vi "SetUpDigi 12bit.vi"(6 "Therapy (T)":bool, 7 "Therapy VISA session in":refnum<visa-resource-name>, 8 "33250(T)/33120(F)":bool=TRUE, 10 "Trigger\nDC (T) AC (F)":bool, 11 "Acqiris ID":u32) -> (0 "Waveform\nGraph":cluster{i32, dbl, dbl[]}(graph), 1 "Equivalent RT delay\ndistance (mm)":dbl=1.5 format="%.4f", 2 "RF data Out":T3 {"Delay (micro s)" format="%.2f"}, 3 "Vert Settings":cluster{u16, i32, "Coupling":u16})   [LabVIEW 2022 SP3]
uses:
  Motion Controllers/-MotionRoutines/MotionGlobals.vi
  <vilib>/Analysis/NI_AALPro.lvlib
  <vilib>/Utility/file.llb/Write To Spreadsheet File (DBL).vi
  <vilib>/Analysis/NI_AALBase.lvlib
  <vilib>/Analysis/baseanly.llb/Mean (DBL).vi
panel:
  in  "LeCroy Path":u16(ring) items=["Pan T/R", "Pan Rec", "Miteq"]
  in  "Cytec T/R":u32
  in  "Panametrics P/R?":bool=TRUE
  in  "Board ID":T1=1 min=1 max=32 step=1
  in  "Save trace?":bool
  out "Lines in burst":i32=1 min=1 max=50000 step=1
  in  "cycles (f), time(t)":bool=TRUE
  in  "Set Panametrics":bool
  out "Total Delay (ms)":dbl=1.5 format="%.2f"
  in  "go to scan type":bool
  in  "Therapy Burst Set Up":T2={"Therapy Set Up"={"Burst time (ms)"=1.0, "Frequency (MHz)"=1.0, "Amplitude (mV)"=10.0}, "Divide prf by"=1, "Therapy Delay (ms) "=0.0, "Turn off therapy (T)"=TRUE} {"Therapy Delay (ms)" format="%.2f"; "Therapy Set Up"."Amplitude (mV)" min=10.0 max=1000.0 format="%.2f"; "Therapy Set Up"."Frequency (MHz)" format="%.4f"; "Therapy Set Up"."Burst time (ms)" min=1 max=50000 step=1 format="%.3f"}
  in  "ExitSendCmd":bool
  in  "Coupling":u16(ring)=2 items=["DC 1 MOhm", "AC 1 MOhm", "DC 50 Ohm", "AC 50 OHM"]
  in  "Voltage Scale":u16(ring)=2
  in  "Time scale per Div":i32(ring)=5 items=["100 ns", "200 ns", "500 ns", "1 micros", "2 micros", "5 micros", "10 micros", "20 micros", "50 micros", "100 micros", "200 micros", "500 micros", "1 ms", "2 ms", "5 ms", "10 ms", "20 ms", "50 ms", "100 ms", "200 ms"]
  out "dup id":i32
  out "Error Message":string
  in  "Trigger Settings":T4={"Source"=2, "Coupling"=0, "Slope"=0, "Level (mV)"=2000.0} {"Slope" items=["Positive", "Negative"]; "Level (mV)" format="%.2f"; "Coupling" items=["DC 1 MOhm", "AC 1 MOhm", "DC 50 Ohm", "AC 50 Ohm"]; "Source" items=["Chan 1", "Chan 2", "External"]}
  in  "RF data Sampling":T5={"Sampling Rate"=0, "Ref Delay (ms)"=0.0, "rf points per line"=2048} {"Ref Delay (ms)" format="%.2f"}
  # "Digitizer Settings"
  # "Scale Settings"
  # "Need to autoscale if viewing spectrum. Yellow curser used for additional delay.\nRF data is captured between yellow and red lines."
  # "© 2000-2002 Riverside Research Institute"
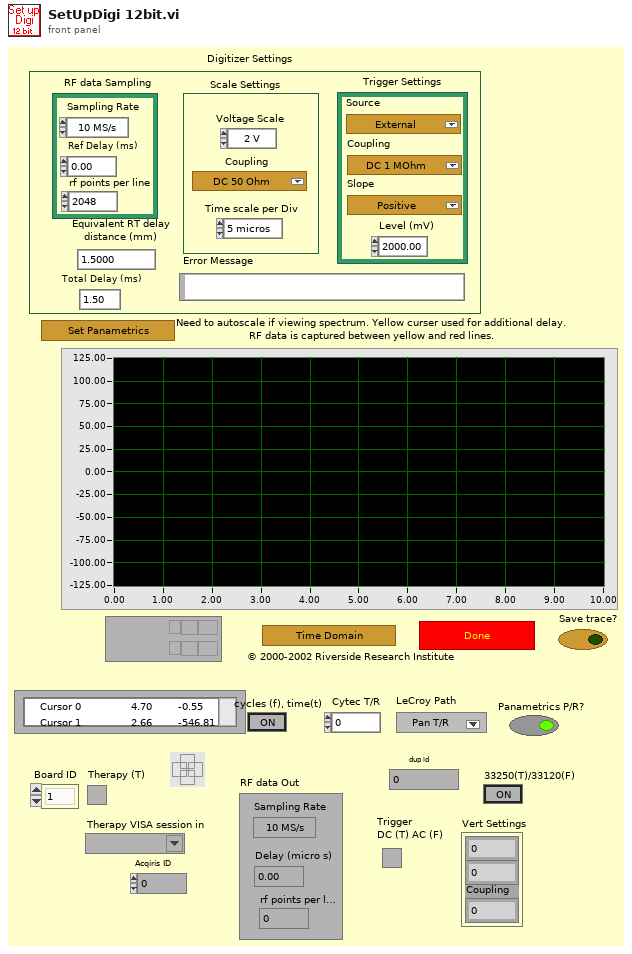
[diagram p1: front panel]
types:
  T1 = typedef "Board Id" = u8
  T2 = cluster{"Therapy Set Up":cluster{"Burst time (ms)":sgl, "Frequency (MHz)":dbl, "Amplitude (mV)":dbl}, "Divide prf by":i32, "Therapy Delay (ms) ":dbl, "Turn off therapy (T)":bool}
  T3 = cluster{"Sampling Rate":u16, "Delay (micro s)":dbl, "rf points per line":u16}
  T4 = cluster{"Source":u16, "Coupling":u16, "Slope":u16, "Level (mV)":dbl}
  T5 = cluster{"Sampling Rate":u16, "Ref Delay (ms)":dbl, "rf points per line":u16}
  T6 = typedef "location.ctl" = enum16{"Automatic", "WCM Main", "Hawaii", "Columbia MM3000", "Columbia  NI System", "NYU", "RRI 2", "UHI Allen", "CUMC RT", "Chiba", "Stony Brook", "WCM Microscopy", "WCM Aeoretch", "WCM Optics Lab", "WCM Main 2Axis", "WCM Rotation", "WCM SAM SMAC", "SERI GP"}
  T7 = cluster{"Burst time (ms)":sgl, "Frequency (MHz)":dbl, "Amplitude (mV)":dbl}
  T8 = cluster{"Voltage Scale":u16, i32, "Coupling":u16}
  T9 = cluster{"returnedSamplesPerSeg":i32, "AddrFirstPoint":i32, "SampTime":dbl, "VGain":dbl, "VOffset":dbl, "NbrSegments":i32, "NbrAvgWforms":i32, "reserved1":dbl, "reserved2":dbl, "reserved3":dbl}
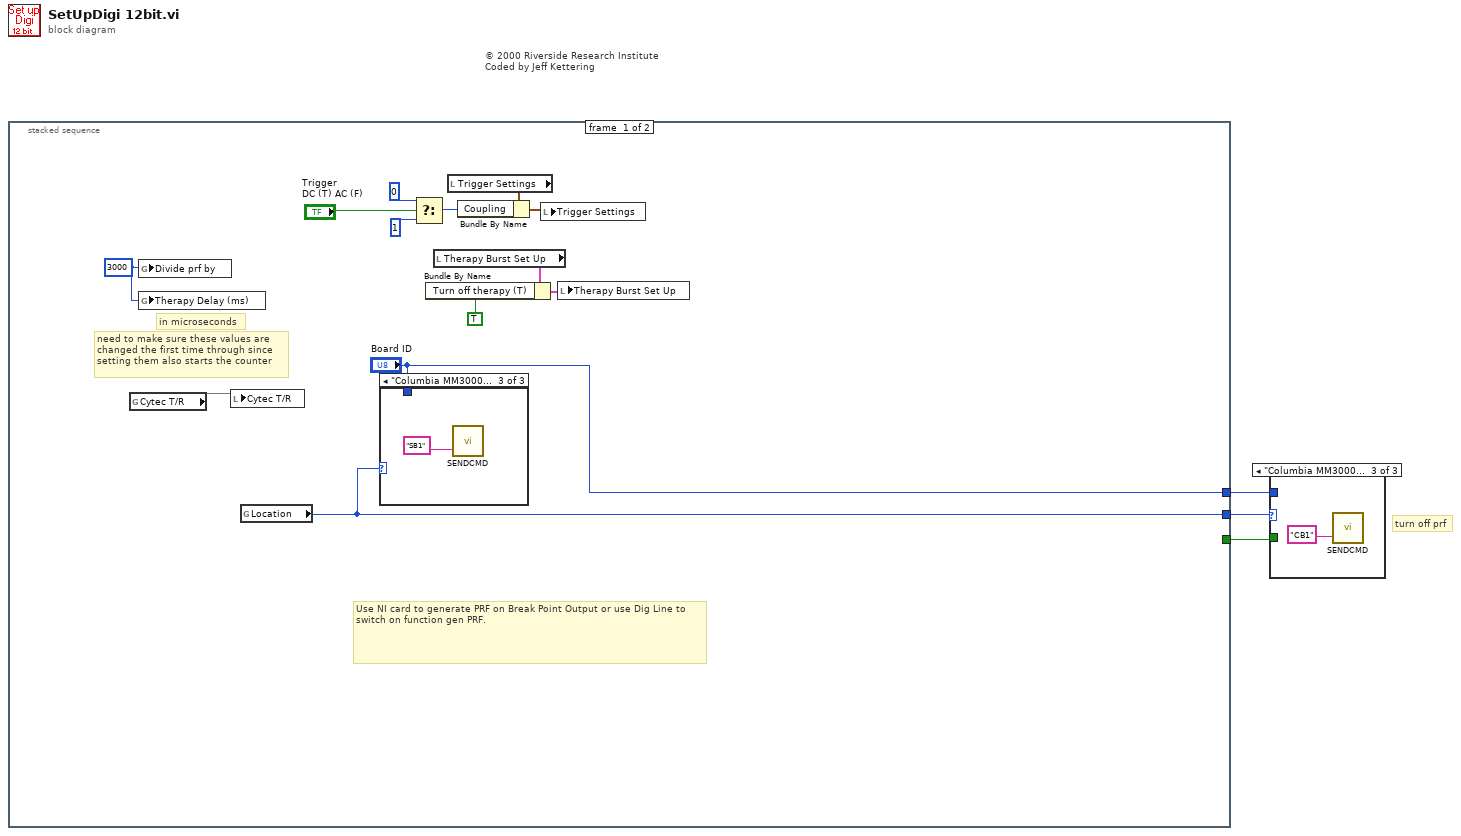
[diagram p0: block diagram]
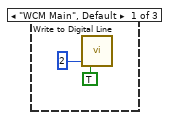
[diagram p2: hidden frame]
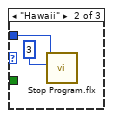
[diagram p3: hidden frame]
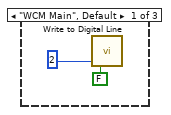
[diagram p4: hidden frame]
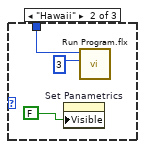
[diagram p5: hidden frame]
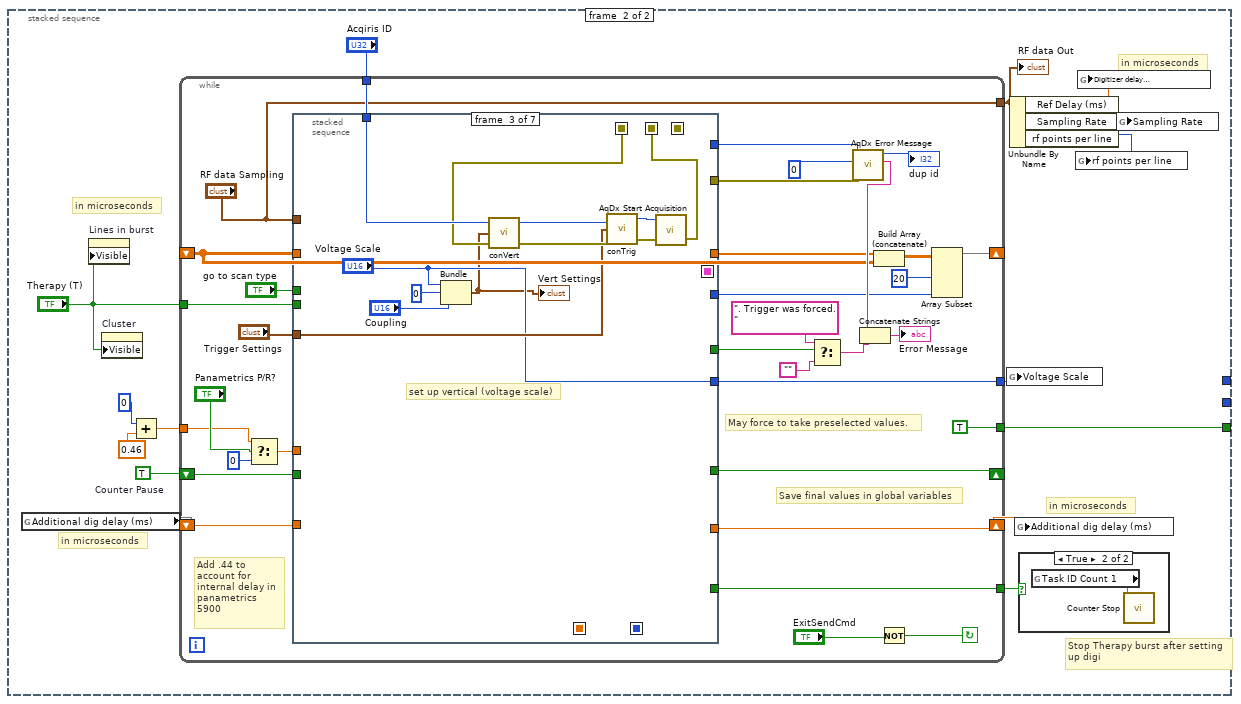
[diagram p6: hidden frame]
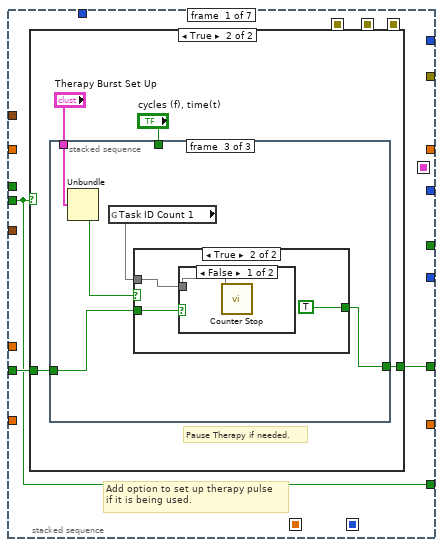
[diagram p7: hidden frame]
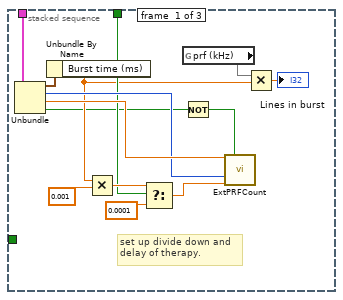
[diagram p9: hidden frame]
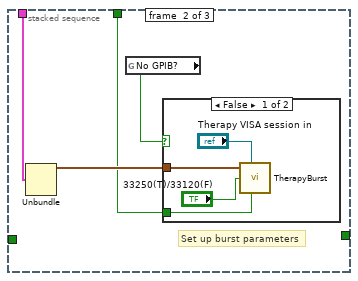
[diagram p10: hidden frame]
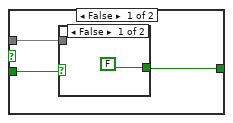
[diagram p12: hidden frame]
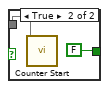
[diagram p13: hidden frame]
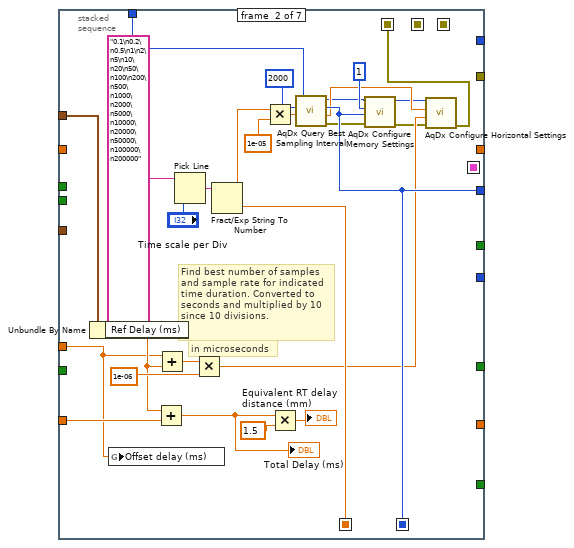
[diagram p15: hidden frame]
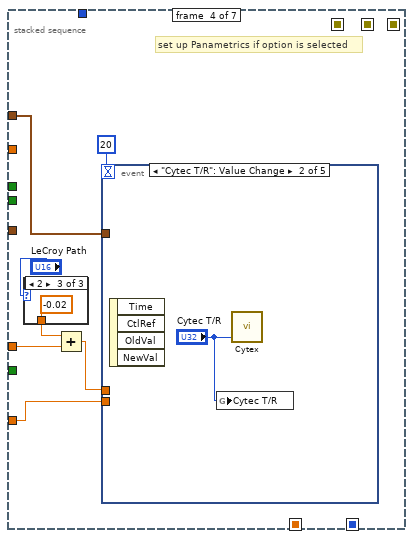
[diagram p16: hidden frame]
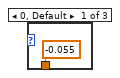
[diagram p17: hidden frame]
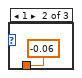
[diagram p18: hidden frame]
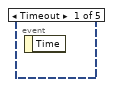
[diagram p19: hidden frame]
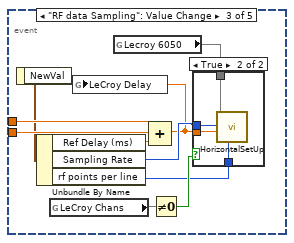
[diagram p20: hidden frame]
diagram:
  # "turn off prf"
  # "© 2000 Riverside Research Institute\nCoded by Jeff Kettering"
  n1 = stacked-sequence {
    tunnel: [w5 _] -> w3
    tunnel: [_ w27] -> w2
    tunnel: ["Board ID" _] -> w1
    frame #0 {
      w10 = 3000
      # "Use NI card to generate PRF on Break Point Output or use Dig Line to switch on function gen PRF."
      # "in microseconds"
      # "need to make sure these values are\nchanged the first time through since\nsetting them also starts the counter"
      n2 = global read "MotionGlobals.vi" "Cytec T/R"() -> (w4)
      n3 = global write "MotionGlobals.vi" "Divide prf by"(w10) -> ()
      n4 = global write "MotionGlobals.vi" "Therapy Delay (ms)"(w10) -> ()
      n5 = local write "Cytec T/R"(w4) -> ()
      n6 = global read "MotionGlobals.vi" "Location"() -> (w5:T6)
      n7 = case shown="\"Columbia MM3000\"" w5 {
        tunnel: "Board ID" -> [_ w20 _]
        frame "WCM Main", Default {
          n8 = call <vilib>:"Write to Digital Line.vi"("line"=2, "line state"=FALSE) -> ()  [unwired: 7 in]
        }
        frame "Hawaii" {
          n9 = property on="Set Panametrics" class="Bool"("Visible"=FALSE) -> ()  [unwired: 2 in, 2 out]
          n10 = call <vilib>:"Run Program.flx"("Program (1)"=3, "Board ID"=w20) -> ()  [unwired: 4 in, 3 out]
        }
        frame "Columbia MM3000" {
          # "turn on prf"
          n11 = call "SENDCMD.VI"("MM2000 Command (ASCII String)"="SB1") -> ()  [unwired: 2 in, 1 out]
        }
      }
      n12 = Select(t=0, s="Trigger\nDC (T) AC (F)", f=1) -> (s? t:f=w11:i32)
      n13 = local read "Therapy Burst Set Up"() -> (w9:T2)
      n14 = Bundle By Name(cluster=w9, "Turn off therapy (T)"=TRUE) -> (w8:T2)
      n15 = local read "Trigger Settings"() -> (w13:T4)
      n16 = Bundle By Name(cluster=w13, "Coupling"=w11) -> (w12:T4)
      n17 = local write "Trigger Settings"(w12) -> ()
      n18 = local write "Therapy Burst Set Up"(w8) -> ()
    }
    frame #1 {
      w36 = TRUE  # Counter Pause
      # "Stop Therapy burst after setting\nup digi"
      # "in microseconds"
      # "in microseconds"
      # "in microseconds"
      # "in microseconds"
      n19 = global read "MotionGlobals.vi" "Additional dig delay (ms)"() -> (w32)
      n20 = property on="Lines in burst" class="DigNum (strict)"("Visible"="Therapy (T)") -> ()  [unwired: 2 in, 2 out]
      n21 = property on="Cluster" class="Clust (strict)"("Visible"="Therapy (T)") -> ()  [unwired: 2 in, 2 out]
      n22 = Add(x=0, y=0.46) -> (x+y=w23:dbl)
      n23 = while {
        tunnel: [TRUE] -> w27
        tunnel: [w49] -> w29
        tunnel: [w50] -> w30
        shift-left: _ -> [w55]
        shift-right: [w53] -> _
        shift-left: w32 -> [w42]
        shift-right: [w40] -> w31
        tunnel: ["RF data Sampling"] -> w34
        shift-left: w36 -> [w59]
        shift-right: [w58] -> _
        tunnel: "Therapy (T)" -> [w60]
        tunnel: "Acqiris ID" -> [w71]
        tunnel: w23 -> [w38]
        stop <- w61 continue-if-true
        # "Add .44 to account for internal delay in panametrics 5900"
        # "May force to take preselected values."
        # "Save final values in global variables"
        n24 = Select(t=w38, s="Panametrics P/R?", f=0) -> (s? t:f=w41:dbl)
        n25 = stacked-sequence {
          seq-local: [_ w128 _ _ _ _ _] -> [_ _ _ _ _ w216 _]
          seq-local: [_ w135 _ _ _ _ _] -> [_ _ _ _ _ w238 w269]
          seq-local: [_ _ _ _ _ w231 _] -> [_ _ _ _ _ _ w270]
          seq-local: [_ w122 _ _ _ _ _] -> [_ _ w151 _ _ _ _]
          seq-local: [_ _ w145 _ _ _ _] -> [_ _ _ _ w182 _ _]
          seq-local: [_ _ _ _ w181 _ _] -> [_ _ _ _ _ w230 _]
          tunnel: w71 -> [_ w136 w154 _ w185 w243 _]
          tunnel: [_ _ _ _ _ w243 _] -> w70
          tunnel: "RF data Sampling" -> [_ w133 _ w161 _ w233 _]
          tunnel: [_ _ _ _ w183 _ _] -> w64
          tunnel: "Trigger Settings" -> [_ _ w148 _ _ _ _]
          tunnel: w60 -> [w72 _ _ _ _ _ _]
          tunnel: w59 -> [w74 _ _ _ _ _ _]
          tunnel: [w73 _ _ _ _ _ _] -> w58
          tunnel: w42 -> [_ w131 _ w158 _ _ _]
          tunnel: [_ _ _ _ _ w232 _] -> w40
          tunnel: w55 -> [_ _ _ _ _ w235 _]
          tunnel: [_ _ _ _ _ w227 _] -> w56
          tunnel: [_ w128 _ _ _ _ _] -> w52
          tunnel: [_ _ "Voltage Scale" _ _ _ _] -> w50
          tunnel: [w72 _ _ _ _ _ _] -> w49
          tunnel: [_ _ _ _ _ w228 _] -> w47
          tunnel: w41 -> [_ w117 _ w160 _ _ _]
          tunnel: "go to scan type" -> [_ _ _ _ _ w220 w268]
          frame #0 {
            # "Add option to set up therapy pulse\nif it is being used."
            n26 = case shown="True" w72 {
              tunnel: w74 -> [w75 w78]
              tunnel: [w75 w77] -> w73
              frame False {
              }
              frame True {
                # "Pause Therapy if needed."
                n27 = stacked-sequence {
                  tunnel: "Therapy Burst Set Up" -> [w85 w97 w103]
                  tunnel: w78 -> [_ _ w105]
                  tunnel: [_ _ w104] -> w77
                  tunnel: "cycles (f), time(t)" -> [w84 w94 _]
                  frame #0 {
                    # "set up divide down and\ndelay of therapy."
                    n28 = Unbundle(w85) -> ("Therapy Set Up"=w91:T7, "Divide prf by"=w92:i32, "Therapy Delay (ms)"=w93:dbl, "Turn off therapy (T)"=w81:bool)
                    n29 = Unbundle By Name(w91) -> ("Burst time (ms)"=w83:sgl)
                    n30 = Multiply(x=w83, y=0.001) -> (x*y=w88:dbl)
                    n31 = Select(t=w88, s=w84, f=0.0001) -> (s? t:f=w90:dbl)
                    n32 = global read "MotionGlobals.vi" "prf (kHz)"() -> (w86)
                    n33 = Not(x=w81) -> (.not. x?=w80:bool)
                    n34 = call "ExtPRFCount.vi"("Therapy Delay (ms)"=w93, "Start Counter?"=w80, "Divide prf by"=w92, "pulse width (s or cycles)"=w90) -> ()  [unwired: 10 in, 2 out]
                    n35 = Multiply(x=w86, y=w83) -> (x*y=→"Lines in burst":sgl)
                  }
                  frame #1 {
                    # "Set up burst parameters"
                    n36 = Unbundle(w97) -> ("Therapy Set Up"=w96:T7)  [unwired: 3 out]
                    n37 = global read "MotionGlobals.vi" "No GPIB?"() -> (w95:bool)
                    n38 = case shown="False" w95 {
                      tunnel: w96 -> [w101 _]
                      tunnel: w94 -> [w100 _]
                      frame False {
                        n39 = call "TherapyBurst.vi"("Input Cluster"=w101, "VISA session in"="Therapy VISA session in", "33250(T)/33120(F)"="33250(T)/33120(F)", "Trigger (F) Gate(T)"=w100) -> ()  [unwired: 2 in, 3 out]
                      }
                      frame True {
                      }
                    }
                  }
                  frame #2 {
                    n40 = Unbundle(w103) -> ("Turn off therapy (T)"=w102:bool)  [unwired: 3 out]
                    n41 = global read "MotionGlobals.vi" "Task ID Count 1"() -> (w106)
                    n42 = case shown="True" w102 {
                      tunnel: w106 -> [w108 w115]
                      tunnel: w105 -> [w109 w113]
                      tunnel: [w107 TRUE] -> w104
                      frame False {
                        n43 = case shown="False" w109 {
                          tunnel: [FALSE FALSE] -> w107
                          tunnel: w108 -> [_ w111]
                          frame False {
                          }
                          frame True {
                            n44 = call <vilib>:"Counter Start.vi"("taskID"=w111) -> ()  [unwired: 9 in, 2 out]
                          }
                        }
                      }
                      frame True {
                        n45 = case shown="False" w113 {
                          tunnel: w115 -> [w116 _]
                          frame False {
                            n46 = call <vilib>:"Counter Stop.vi"("taskID"=w116) -> ()  [unwired: 5 in, 2 out]
                          }
                          frame True {
                          }
                        }
                      }
                    }
                  }
                }
              }
            }
          }
          frame #1 {
            # "in microseconds"
            # "Find best number of samples\nand sample rate for indicated\ntime duration. Converted to\nseconds and multiplied by 10\nsince 10 divisions."
            n47 = Unbundle By Name(w133) -> ("Ref Delay (ms)"=w119:dbl)
            n48 = global write "MotionGlobals.vi" "Offset delay (ms)"(w117) -> ()
            n49 = Add(x=w119, y=w131) -> (x+y=w118:dbl)
            "Total Delay (ms)" <- w118
            n50 = Add(x=w117, y=w119) -> (x+y=w120:dbl)
            n51 = Pick Line(multi-line string="0.1\n0.2\n0.5\n1\n2\n5\n10\n20\n50\n100\n200\n500\n1000\n2000\n5000\n10000\n20000\n50000\n100000\n200000" ("ResourceName"), line index="Time scale per Div") -> (output string=w142:string)  [unwired: 1 in]
            n52 = Multiply(x=w120, y=1e-06) -> (x*y=w127:dbl)
            n53 = Fract/Exp String To Number(string=w142) -> (number=w135:dbl)  [unwired: 3 in, 1 out]
            n54 = Multiply(x=w135, y=1e-05) -> (x*y=w140:dbl)
            n55 = Multiply(x=w118, y=1.5) -> (x*y=→"Equivalent RT delay\ndistance (mm)":dbl)
            n56 = call "AqDx Query Best Sampling Interval.vi"("Time Window (1E-6 s)"=w140, "Maximum Samples (10000)"=2000, "Instrument ID"=w136) -> ("error out"=w121:errorcluster, "Sampling Interval (s)"=w126:dbl, "Nominal Samples"=w128:i32, "dup Instrument ID"=w125:u32)  [unwired: 1 in]
            n57 = call "AqDx Configure Memory Settings.vi"("error in (no error)"=w121, "Number of Samples (1000)"=w128, "Number of Segments (1)"=1, "Instrument ID"=w125) -> ("error out"=w123:errorcluster, "dup Instrument ID"=w124:u32)  [unwired: 2 in]
            n58 = call "AqDx Configure Horizontal Settings.vi"("error in (no error)"=w123, "Delay Time (0 s)"=w127, "Sampling Interval (10 ns)"=w126, "Instrument ID"=w124) -> ("error out"=w122:errorcluster)  [unwired: 2 in, 1 out]
          }
          frame #2 {
            # "set up vertical (voltage scale)"
            n59 = Bundle("Voltage Scale"="Voltage Scale", 0, "Coupling"="Coupling") -> (w143:T8)  [unwired: 1 in]
            "Vert Settings" <- w143
            n60 = call "conVert.vi"("InstrumentID"=w154, "V scale"=w143, "error in"=w151) -> ("Status"=w149:i32, "error out"=w150:errorcluster)  [unwired: 3 in]
            n61 = call "conTrig.vi"("error in"=w150, "Trigger"=w148, "InstrumentID"=w149) -> ("error out"=w147:errorcluster, "dup id"=w146:i32)  [unwired: 1 in]
            n62 = call "AqDx Start Acquisition.vi"("error in (no error)"=w147, "Instrument ID"=w146) -> ("error out"=w145:errorcluster)  [unwired: 1 in, 1 out]
          }
          frame #3 {
            # "set up Panametrics if option is selected"
            n63 = case shown="2" "LeCroy Path" {
              tunnel: [-0.055 -0.06 -0.02] -> w156
              frame 0, Default {
              }
              frame 1 {
              }
              frame 2 {
              }
            }
            n64 = Add(x=w156, y=w160) -> (x+y=w159:dbl)
            n65 = event shown="[1] \"Cytec T/R\": Value Change" {
              selector: _ -> [_ _ _ _ _]
              dyn-events: _ -> [_ _ _ _ _]
              timeout: 20 -> [_ _ _ _ _]
              tunnel: w158 -> [_ _ w171 _ _]
              tunnel: w161 -> [_ _ _ w180 _]
              tunnel: w159 -> [_ _ w170 _ _]
              event Timeout {
                n66 = event-data() -> ()  [unwired: 1 in, 1 out]
              }
              event "Cytec T/R": Value Change {
                n67 = event-data() -> ()  [unwired: 1 in, 4 out]
                n68 = global write "MotionGlobals.vi" "Cytec T/R"("Cytec T/R") -> ()
                n69 = call "Cytex.vi"("Xmit Ring"="Cytec T/R") -> ()  [unwired: 1 in, 2 out]
              }
              event "RF data Sampling": Value Change {
                n70 = event-data() -> ("NewVal"=w166:T5)  [unwired: 1 in]
                n71 = Unbundle By Name(w166) -> ("Ref Delay (ms)"=w172:dbl, "Sampling Rate"=w168:u16, "rf points per line"=w169:u16)
                n72 = global read "MotionGlobals.vi" "LeCroy Chans"() -> (w174)
                n73 = global read "MotionGlobals.vi" "Lecroy 6050"() -> (w175)
                n74 = Compound Arithmetic op=ADD(w170, w171, w172) -> (w167:dbl)
                n75 = global write "MotionGlobals.vi" "LeCroy Delay"(w167) -> ()
                n76 = Not Equal To 0?(x=w174) -> (x != 0?=w173:bool)
                n77 = case shown="True" w173 {
                  tunnel: w167 -> [_ w179]
                  tunnel: w175 -> [_ w178]
                  tunnel: w169 -> [_ w177]
                  tunnel: w168 -> [_ w176]
                  frame False {
                  }
                  frame True {
                    n78 = call "HorizontalSetUp.vi"("ActXDSO In"=w178, "Sampling Rate"=w176, "Delay (micsec)"=w179, "rf points"=w177) -> ()  [unwired: 1 in, 2 out]
                  }
                }
              }
              event "Waveform\nGraph": Mouse Up {
                n79 = event-data() -> ()  [unwired: 1 in, 1 out]
                n80 = property on="RF data Sampling" class="Clust (strict)"("Value (Signaling)"=w180) -> ()  [unwired: 2 in, 2 out]
              }
              event "Set Panametrics": Value Change {
                # "set up Panametrics if option is selected"
                n81 = event-data() -> ()  [unwired: 1 in, 6 out]
                n82 = call "5900PRSet.vi"() -> ()  [unwired: 13 in, 3 out]
              }
            }
          }
          frame #4 {
            # "wait for end of acquistion"
            n83 = Tick Count (ms)() -> (millisecond timer value=w186:u32)
            n84 = while {
              shift-left: FALSE -> [w195]
              shift-right: [w196] -> w183
              shift-left: w186 -> [w199]
              shift-right: [w200] -> _
              tunnel: w185 -> [w192]
              tunnel: w182 -> [w193]
              tunnel: [w189] -> w181
              stop <- w198 stop-if-true
              n85 = Tick Count (ms)() -> (millisecond timer value=w204:u32)
              n86 = call "AqDx Query Acquisition Status.vi"("error in (no error)"=w193, "Instrument ID"=w192) -> ("error out"=w190:errorcluster, "Done?"=w194:bool, "dup Instrument ID"=w191:u32)  [unwired: 2 in, 1 out]
              n87 = Unbundle(w190) -> ("status"=w188:bool)  [unwired: 2 out]
              n88 = Subtract(x=w204, y=w199) -> (x-y=w202:u32)
              n89 = Or(x=w194, y=w188) -> (x .or. y?=w197:bool)
              n90 = Greater?(x=w202, y=1000) -> (0:w203:bool)
              n91 = case shown="True" w203 {
                tunnel: w191 -> [_ w214]
                tunnel: [w208 w213] -> w200
                tunnel: w199 -> [w208 _]
                tunnel: [w207 w212] -> w198
                tunnel: w197 -> [w207 w212]
                tunnel: [w206 TRUE] -> w196
                tunnel: w195 -> [w206 _]
                tunnel: w190 -> [w205 w210]
                tunnel: [w205 w209] -> w189
                frame False {
                }
                frame True {
                  n92 = Tick Count (ms)() -> (millisecond timer value=w213:u32)
                  n93 = call "AqDx Software Trigger.vi"("error in (no error)"=w210, "Instrument ID"=w214) -> ("error out"=w209:errorcluster)  [unwired: 1 in, 1 out]
                }
              }
              n94 = Wait (ms)(milliseconds to wait=10) -> ()  [unwired: 1 out]
            }
          }
          frame #5 {
            w236 = u32 1 ("Write Attribute")
            # "Can View Spectrum Also"
            # "Read voltage and convery to MV. Make plot\nshowing what will be captured as RF data. Yellow\ncurser can be moved to provide addtional time shift for digitizer\ndealy."
            n95 = property on="Waveform Graph" class="WFGraph (strict)"("Active Cursor"=w236) -> ("Cursor.Cursor Position:Cursor X"=w239:dbl)  [unwired: 2 in, 2 out]
            n96 = Divide(x=10, y=w216) -> (x/y=w223:dbl)
            n97 = Multiply(x=w216, y=w216) -> (x*y=w221:i32)
            n98 = call "GetWaveform.vi"("Read Mode"=enum32{"ADC", "Volts"}."Volts", "error in"=w230, "Num Segs"=1, "Num Samps"=w216, "Acq ID Out"=w243) -> ("error out"=w228:errorcluster, "first row"=w215:dbl[], "dataDesc"=w219:T9)  [unwired: 1 in, 3 out]
            n99 = Less Than 0?(x=w239) -> (x < 0?=w237:bool)
            n100 = Unbundle By Name(w219) -> ("SampTime"=w229:dbl)
            n101 = case shown="True" w237 {
              tunnel: w239 -> [w245 _]
              tunnel: [w245 w246] -> w225
              tunnel: w236 -> [_ w248]
              frame False {
              }
              frame True {
                w246 = 0
                n102 = property on="Waveform Graph" class="WFGraph (strict)"("X Scale.Range:Minimum"=w246, "X Scale.Range:Maximum"=10, "Active Cursor"=w248, "Cursor.Cursor Position:Cursor X"=w246) -> ()  [unwired: 2 in, 2 out]
              }
            }
            n103 = case shown="True" w220 {
              tunnel: [w251 w263] -> w234
              tunnel: w215 -> [w250 w259]
              tunnel: [w252 w255] -> w240
              tunnel: w223 -> [w252 _]
              tunnel: w235 -> [_ w258]
              tunnel: w229 -> [_ w257]
              tunnel: [i32[] [] w254] -> w227
              tunnel: w221 -> [_ _]
              frame False {
                n104 = Multiply(x=w250, y=1000) -> (x*y=w251:dbl[])
              }
              frame True {
                n105 = Transpose 2D Array(2D array=w258) -> (transposed array=w260:dbl[][])
                n106 = for {
                  tunnel: w260 -> [w267] mode=indexing
                  tunnel: [w266] -> w261 mode=indexing
                  n107 = call-poly <vilib>:"Mean.vi"("X"=w267) -> ("mean"=w266:dbl)  [unwired: 1 out]
                }
                n108 = call <vilib>:"Auto Power Spectrum.vi"("dt"=w257, "Signal (V)"=w259) -> ("df"=w256:dbl, "Power Spectrum (V^2 rms)"=w254:dbl[])
                n109 = Multiply(x=w256, y=1e-06) -> (x*y=w255:dbl)
                n110 = Logarithm Base 10(1:w261) -> (0:w264:dbl[])
                n111 = Multiply(x=10, y=w264) -> (x*y=w263:dbl[])
              }
            }
            n112 = call "RFWindow.vi"("RF data Sampling"=w233, "Sample Time"=w229) -> ("curser position"=w222:dbl)  [unwired: 2 in]
            n113 = Multiply(x=w223, y=w222) -> (x*y=w226:dbl)
            n114 = Add(x=w226, y=w225) -> (x+y=w224:dbl)
            n115 = property on="Waveform Graph" class="WFGraph (strict)"("Active Cursor"=0, "Cursor.Cursor Position:Cursor X"=w224) -> ()  [unwired: 2 in, 2 out]
            n116 = Bundle(0, w240, w234) -> (w231:cluster{i32, dbl, dbl[]})  [unwired: 1 in]
            n117 = Multiply(x=w225, y=w238) -> (x*y=w232:dbl)
          }
          frame #6 {
            n118 = case shown="True" "Save trace?" {
              tunnel: w270 -> [_ w282]
              tunnel: w269 -> [_ w275]
              tunnel: w268 -> [_ w273]
              frame False {
              }
              frame True {
                n119 = Unbundle(w282) -> (w281:dbl, w280:dbl[])  [unwired: 1 out]
                n120 = for {
                  tunnel: w281 -> [w284]
                  tunnel: w280 -> [_] mode=indexing
                  tunnel: [w283] -> w277 mode=indexing
                  i -> [w285]
                  n121 = Multiply(x=w284, y=w285) -> (x*y=w283:dbl)
                }
                n122 = Select(t=1, s=w273, f=w275) -> (s? t:f=w272:dbl)
                n123 = Multiply(x=w277, y=w272) -> (x*y=w276:dbl[])
                n124 = Build Array(w276, w280) -> (w279:dbl[][])
                n125 = Transpose 2D Array(2D array=w279) -> (transposed array=w278:dbl[][])
                n126 = call-poly <vilib>:"Write To Spreadsheet File.vi"("2D data"=w278) -> ()  [unwired: 7 in, 1 out]
              }
            }
            "Waveform\nGraph" <- w270
          }
        }
        n127 = Select(t=". Trigger was forced.", s=w64, f="") -> (s? t:f=w66:string)
        n128 = call "AqDx Error Message.vi"("Instrument ID"=w70, "Type of Dialog (1: OK Msg)"=0, "error in (no error)"=w47) -> ("dup Instrument ID"=→"dup id":u32, "Error Message"=w69:string)  [unwired: 2 in, 3 out]
        n129 = Concatenate Strings(w69, w66) -> (→"Error Message":string)
        n130 = Build Array (concatenate)(w56, w55) -> (w54:dbl[][])
        n131 = Not(x="ExitSendCmd") -> (.not. x?=w61:bool)
        n132 = Array Subset(array=w54, length (row)=20, length (col)=w52) -> (w53:dbl[][])  [unwired: 2 in]
      }
      "RF data Out" <- w34
      n133 = global write "MotionGlobals.vi" "Voltage Scale"(w30) -> ()
      n134 = Unbundle By Name(w34) -> ("Ref Delay (ms)"=w26:dbl, "Sampling Rate"=w35:u16, "rf points per line"=w33:u16)
      n135 = global write "MotionGlobals.vi" "Additional dig delay (ms)"(w31) -> ()
      n136 = case shown="True" w29 {
        frame False {
        }
        frame True {
          n137 = global read "MotionGlobals.vi" "Task ID Count 1"() -> (w286)
          n138 = call <vilib>:"Counter Stop.vi"("taskID"=w286) -> ()  [unwired: 5 in, 2 out]
        }
      }
      n139 = global write "MotionGlobals.vi" "rf points per line"(w33) -> ()
      n140 = global write "MotionGlobals.vi" "Digitizer delay\n (ms)"(w26) -> ()
      n141 = global write "MotionGlobals.vi" "Sampling Rate"(w35) -> ()
    }
  }
  n142 = case shown="\"Columbia MM3000\"" w3 {
    tunnel: w2 -> [_ _ _]
    tunnel: w1 -> [_ w289 _]
    frame "WCM Main", Default {
      n143 = call <vilib>:"Write to Digital Line.vi"("line"=2, "line state"=TRUE) -> ()  [unwired: 7 in]
    }
    frame "Hawaii" {
      n144 = call <vilib>:"Stop Program.flx"("Program (1)"=3, "Board ID"=w289) -> ()  [unwired: 4 in, 3 out]
    }
    frame "Columbia MM3000" {
      n145 = call "SENDCMD.VI"("MM2000 Command (ASCII String)"="CB1") -> ()  [unwired: 2 in, 1 out]
    }
  }
